vi "ESP301_STOP.vi"(10 "axisNumber":i32=1, 11 "COM_PORT":string="COM12") -> (0 "errstring":string, 8 "Error":bool)   [LabVIEW 2019]
uses:
  Newport.ESP301.CommandInterface
panel:
  out "MO_Set":i32
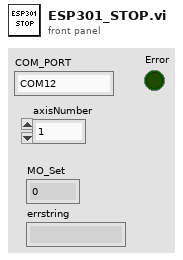
[diagram p1: front panel]
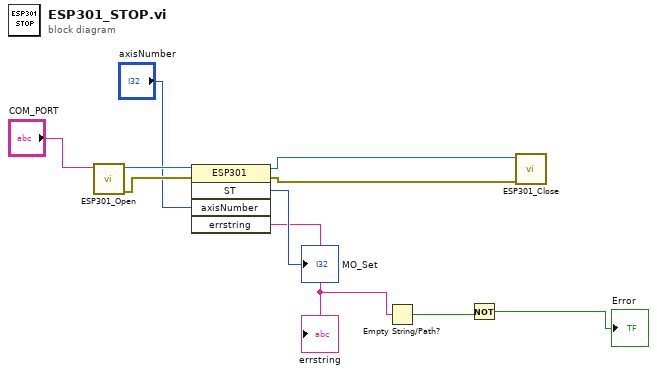
[diagram p0: block diagram]
diagram:
  n1 = call "ESP301_Open.vi"("strDeviceKey"="COM_PORT") -> ("sortie d'erreur"=w9:errorcluster, "référence en sortie"=w10:refnum<k24>)  [unwired: 9 in]
  n2 = invoke on="Nœud de méthode" class="ESP301" method="ST"(reference=w10, error in=w9, "axisNumber"="axisNumber") -> (reference out=w6:refnum<k24>, error out=w5:errorcluster, "ST"=→"MO_Set":i32, "errstring"=w3:string)  [unwired: 2 in, 1 out]
  "errstring" <- w3
  n3 = Empty String/Path?(string/path=w3) -> (empty?=w2:bool)
  n4 = Not(x=w2) -> (.not. x?=→"Error":bool)
  n5 = call "ESP301_Close.vi"("entrée d'erreur (pas d'erreur)"=w5, "référence"=w6) -> ()  [unwired: 9 in, 1 out]
